vi "Read Configuration.vi"(8 "error in (no error)":errorcluster, 11 "Execution UI In":refnum<class "Execution UI.lvclass">) -> (0 "error out":errorcluster, 3 "Execution UI Out":refnum<class "Execution UI.lvclass">)   [LabVIEW 2020, in "Execution UI.lvclass"]
doc: "Method that read any necessay configurations from config file or potentially configure hard coded values. The specified configuration file is validated and loaded."
uses:
  Execution UI.lvclass
  Application Framework/Support/Configuration File/Configuration File.lvlib
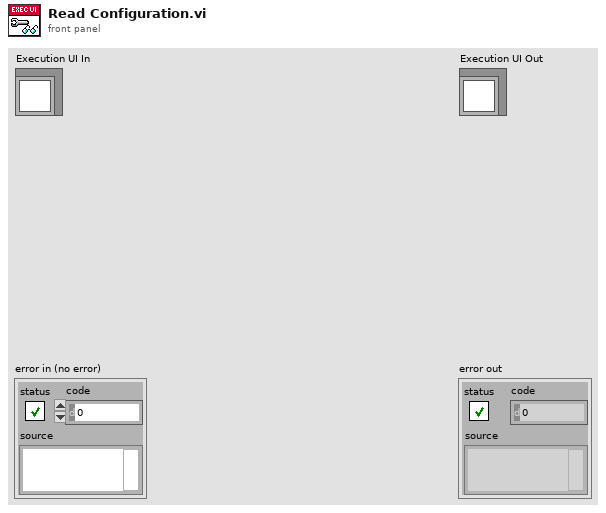
[diagram p1: front panel]
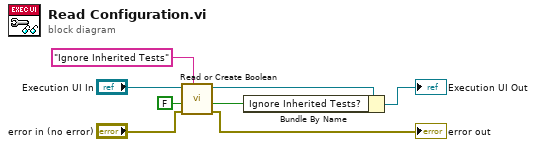
[diagram p0: block diagram]
diagram:
  n1 = call "Read or Create Boolean.vi"("key"="Ignore Inherited Tests", "error in (no error)"="error in (no error)", "default value"=FALSE, "Process in"="Execution UI In") -> ("error out"=→"error out":errorcluster, "value"=w1:bool, "Process out"=w7:refnum<class "Execution UI.lvclass">)  [unwired: 4 in, 1 out]
  n2 = Bundle By Name(cluster=w7, "Ignore Inherited Tests?"=w1) -> (→"Execution UI Out":refnum<class "Execution UI.lvclass">)
